vi "HB_Simple.Main Very Simple Reference.vi"() -> ()   [LabVIEW 2009, in "HB_BaseClass_Examples.lvlib"]
doc: "Simple demo VI."
uses:
  HB_BaseClass_Examples.lvlib
  HB_Simple.lvclass
  lib.lib/HGF_LVC/HGF_Auxiliary/HGF_Auxiliary.lvlib
  lib.lib/HGF_LVC/HGF_BaseClasses/HGF_Reference/HGF_Reference.lvclass
panel:
  out "x 2":dbl
  out "x 1":dbl
  out "success":bool
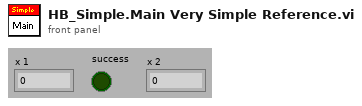
[diagram p1: front panel]
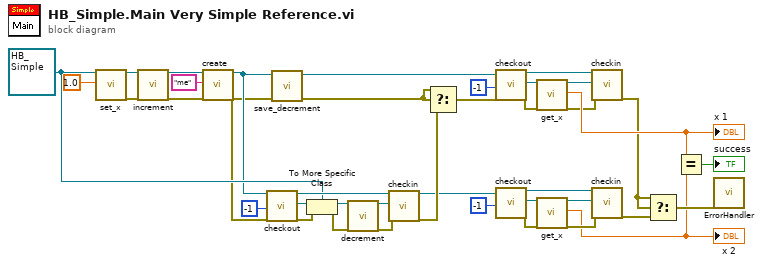
[diagram p0: block diagram]
diagram:
  w16 = refnum<class "HB_Simple.lvclass"> refnum ("HGF_BaseClass_Examples.lvlib:HB_Simple.lvclass")
  n1 = call "set_x.vi"("HB_Simple"=w16, "x"=1.0) -> ("dup HB_Simple"=w38:refnum<class "HB_Simple.lvclass">, "error out"=w37:errorcluster)  [unwired: 1 in, 15 out]
  n2 = call "increment.vi"("HB_Simple in"=w38, "error in (no error)"=w37) -> ("HB_Simple out"=w34:refnum<class "HB_Simple.lvclass">, "error out"=w33:errorcluster)  [unwired: 16 out]
  n3 = call "create.vi"("Object"=w34, "name"="me", "error in (no error)"=w33) -> ("HGF_Reference"=w5:refnum<class "HGF_Reference.lvclass">, "error out"=w4:errorcluster)  [unwired: 15 out]
  n4 = call "checkout.vi"("HGF_Reference"=w5, "timeout in ms (-1)"=-1, "error in (no error)"=w4) -> ("dup HGF_Reference"=w26:refnum<class "HGF_Reference.lvclass">, "Object"=w30:refnum<class>, "error out"=w29:errorcluster)  [unwired: 14 out]
  n5 = call "save_decrement.vi"("error in (no error)"=w4, "HGF_Reference"=w5) -> ("error out"=w2:errorcluster, "dup HGF_Reference"=w3:refnum<class "HGF_Reference.lvclass">)  [unwired: 8 in]
  n6 = To More Specific Class(target class=w16, reference=w30, error in=w29) -> (specific class reference=w27:refnum<class "HB_Simple.lvclass">, error out=w28:errorcluster)
  n7 = call "decrement.vi"("HB_Simple in"=w27, "error in (no error)"=w28) -> ("HB_Simple out"=w24:refnum<class "HB_Simple.lvclass">, "error out"=w25:errorcluster)  [unwired: 16 out]
  n8 = call "checkin.vi"("HGF_Reference"=w26, "Object"=w24, "error in (no error)"=w25) -> ("dup HGF_Reference"=w6:refnum<class "HGF_Reference.lvclass">, "error out"=w7:errorcluster)  [unwired: 1 in, 14 out]
  n9 = Select(t=w2, s=w2, f=w7) -> (s? t:f=w15:errorcluster)
  n10 = call "checkout.vi"("HGF_Reference"=w3, "timeout in ms (-1)"=-1, "error in (no error)"=w15) -> ("dup HGF_Reference"=w20:refnum<class "HGF_Reference.lvclass">, "HB_Simple"=w23:refnum<class "HB_Simple.lvclass">, "error out"=w22:errorcluster)  [unwired: 14 out]
  n11 = call "checkout.vi"("HGF_Reference"=w6, "timeout in ms (-1)"=-1) -> ("dup HGF_Reference"=w12:refnum<class "HGF_Reference.lvclass">, "HB_Simple"=w9:refnum<class "HB_Simple.lvclass">, "error out"=w10:errorcluster)  [unwired: 1 in, 14 out]
  n12 = call "get_x.vi"("HB_Simple"=w23, "error in (no error)"=w22) -> ("dup HB_Simple"=w19:refnum<class "HB_Simple.lvclass">, "x"=w40:dbl, "error out"=w18:errorcluster)  [unwired: 15 out]
  "x 1" <- w40
  n13 = call "get_x.vi"("HB_Simple"=w9, "error in (no error)"=w10) -> ("dup HB_Simple"=w13:refnum<class "HB_Simple.lvclass">, "x"=w1:dbl, "error out"=w14:errorcluster)  [unwired: 15 out]
  "x 2" <- w1
  n14 = call "checkin.vi"("HGF_Reference"=w20, "Object"=w19, "error in (no error)"=w18) -> ("error out"=w17:errorcluster)  [unwired: 1 in, 15 out]
  n15 = call "checkin.vi"("HGF_Reference"=w12, "Object"=w13, "error in (no error)"=w14) -> ("error out"=w8:errorcluster)  [unwired: 1 in, 15 out]
  n16 = Select(t=w17, s=w17, f=w8) -> (s? t:f=w35:errorcluster)
  n17 = Equal?(x=w40, y=w1) -> (x = y?=→"success":bool)
  n18 = call "ErrorHandler.vi"("error in (no error)"=w35) -> ()  [unwired: 6 in, 13 out]
